vi "CreateInterface.vi"(0 "ClassWriter.lvclass":refnum<class "ClassWriter.lvclass">, 1 "ProjectTreePosition(String or Project Item Ref)":variant, 2 "CreateInterfaceData":T1, 5 "error in (no error)":errorcluster, 6 "KeepLvClassRefOpen(False)":bool, 7 "HeaderToApply (take from VIRef or /use 2D-8bit header, Ignored if not wired)":variant) -> (14 "ClassWriter.lvclass":refnum<class "ClassWriter.lvclass">, 15 "LVClassLibraryRefnum":refnum<vi>, 19 "error out":errorcluster)   [LabVIEW 2020, in "ClassWriter.lvclass"]
uses:
  <resource>/Framework/Providers/Open_GDS/ClassProviders/Provider_BaseClassInterface/ClassWriter_class/ClassWriter.lvclass
  <resource>/Framework/Providers/Open_GDS/ClassProviders/Provider_BaseClassInterface/CreateInterfaceData.ctl
  <resource>/Framework/Providers/Open_GDS/ClassProviders/Provider_BaseClassInterface/ClassWriter_class/InterfaceMethodsToCreate.ctl
  <resource>/Framework/Providers/Open_GDS/ClassProviders/Common/CommonVIs/CommonVIs_AttributeType.ctl
  <resource>/Framework/Providers/Open_GDS/ClassProviders/Common/CommonVIs/CommonVIs_AttributeDataType.ctl
  <resource>/Framework/Providers/Open_GDS/ClassProviders/Common/String/GDSString_AccessScopeModifierType.ctl
  <resource>/Framework/Providers/Open_GDS/ClassProviders/Provider_BaseClassInterface/ClassWriter_class/InterfacesToImplement.ctl
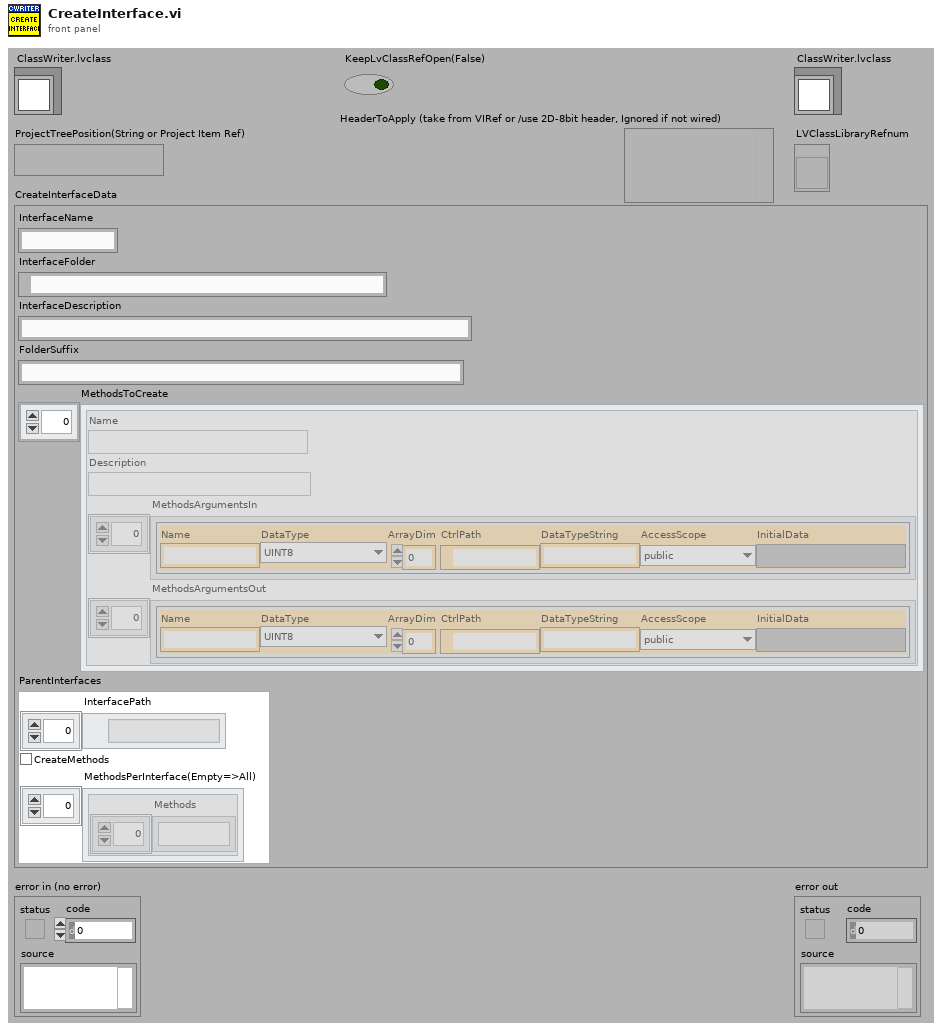
[diagram p1: front panel]
types:
  T1 = typedef "ClassWriter.lvclass/CreateInterfaceData.ctl" = cluster{"InterfaceName":string, "InterfaceFolder":path, "InterfaceDescription":string, "FolderSuffix":string, "MethodsToCreate":T2[], "ParentInterfaces":T6}
  T2 = typedef "ClassWriter.lvclass/InterfaceMethodsToCreate.ctl" = cluster{"Name":string, "Description":string, "MethodsArgumentsIn":T3[], "MethodsArgumentsOut":T3[]}
  T3 = typedef "CommonVIs_AttributeType.ctl" = cluster{"Name":string, "DataType":T4, "ArrayDim":i32, "CtrlPath":path, "DataTypeString":string, "AccessScope":T5, "InitialData":variant}
  T4 = typedef "CommonVIs_AttributeDataType.ctl" = enum16{"UINT8", "INT8", "UINT16", "INT16", "UINT32", "INT32", "UINT64", "INT64", "SGL", "DBL", "EXT", "CSG", "CDB", "CXT", "TimeStamp", "STRING", "PATH", "BOOL", "ENUM", "RefNum", "VIRefNum", "LabVIEW Class", "Cluster", "Variant", "TypeDef", "Waveform", "LabVIEW Object", "Other", "void"}
  T5 = typedef "GDSString_AccessScopeModifierType.ctl" = enum16{"public", "private", "protected", "internal"}
  T6 = typedef "ClassWriter.lvclass/InterfacesToImplement.ctl" = cluster{"InterfacePath":path[], "CreateMethods":bool, "MethodsPerInterface(Empty=>All)":cluster{"Methods":string[]}[]}
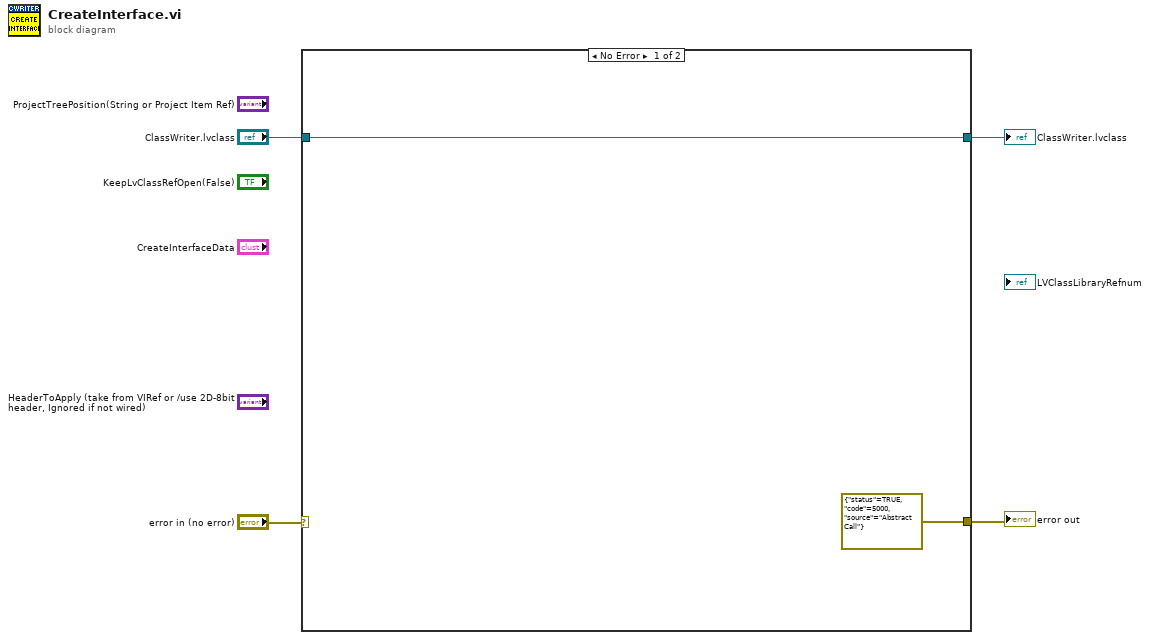
[diagram p0: block diagram]
diagram:
  n1 = case shown="No Error" "error in (no error)" {
    selector: "error in (no error)" -> [_ w7]
    tunnel: "ClassWriter.lvclass" -> [w5 w8]
    tunnel: [errorcluster {"status"=TRUE, "code"=5000, "source"="Abstract Call"} ("error IO") w7] -> w3
    tunnel: [w5 w8] -> w2
    frame No Error {
    }
    frame Error {
    }
  }
  "ClassWriter.lvclass" <- w2
  "error out" <- w3
